vi "test.vi"() -> ()   [LabVIEW 2010, in "Map.lvclass"]
doc: "Test program for the Map class, demonstrating how to use its functionality."
uses:
  Map.lvclass
panel:
  in  "clear button":bool
  in  "delete-element keys":string[](array[string]) caption="key chain"
  in  "delete button":bool
  out "value out":string
  in  "fetch array":bool
  in  "fetch keys":string[](array[string]) caption="key chain"
  in  "insert submap":bool
  in  "insert submap keys":string[](array[string]) caption="key chain"
  in  "insert element":bool
  in  "value in":string
  in  "insert-element keys":string[](array[string]) caption="key chain"
  in  "stop":bool
  in  "elements":string(tree)
  # "Map test program"
  # "The Map class provides the functionality of an associative array, which is a collection of key-value pairs.\n\nYou can address individual elements (values) of a map using a unique key (a string). \n\nAny data type is supported as a value. In this test program only strings and (sub-)Maps are used as values, however.\n\nNested maps (tree-like structures) are possible because a Map can itself be used as a value. You can access values (either submaps or terminal nodes) in the hierarchy by means of key chains (a key chain is an array of strings).\n\nInvidiual elements (nodes) can be added to the tree hierarchy even if parent nodes do not yet exist: just provide a key chain and missing nodes are generated on the fly."
  # "Assign element"
  # "Assign submap"
  # "Fetch element"
  # "Delete element/submap"
  # "Clear map"
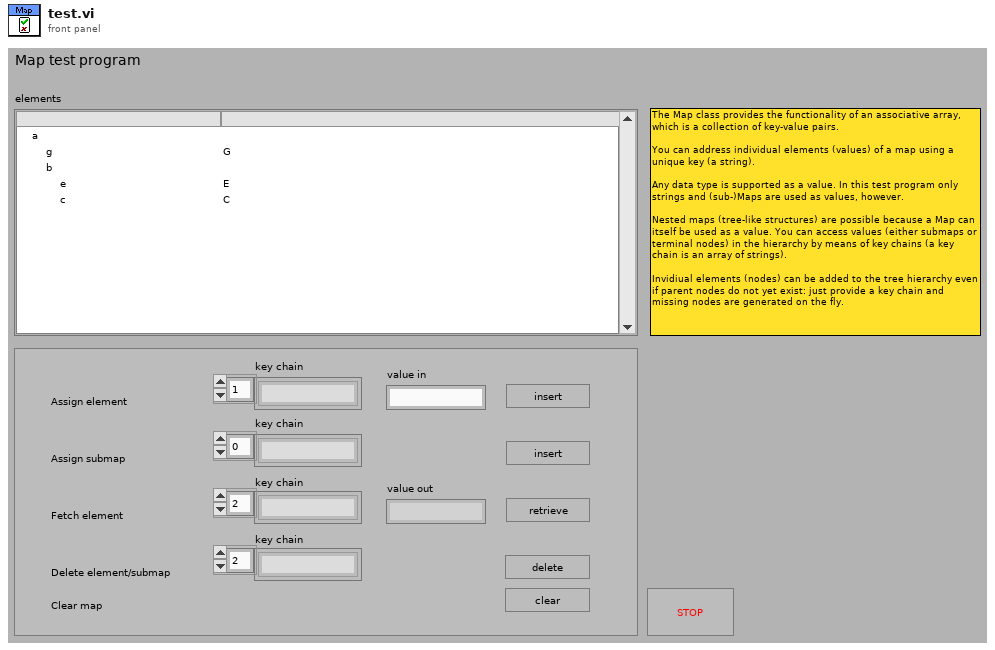
[diagram p1: front panel]
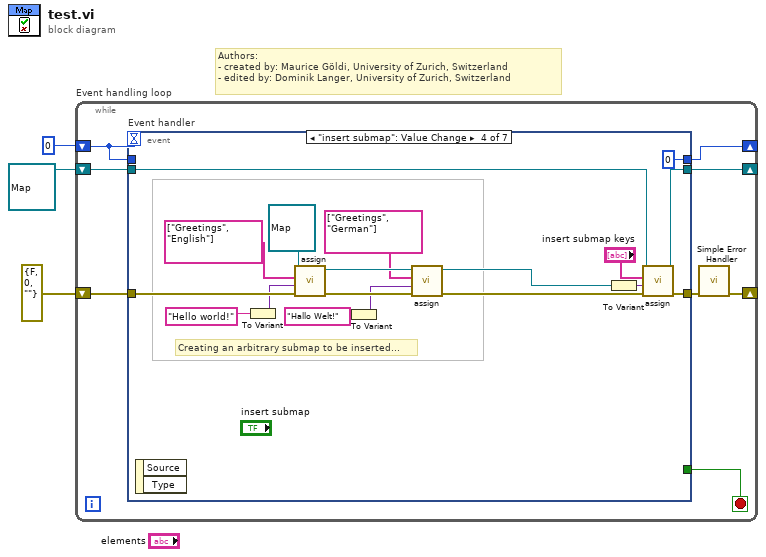
[diagram p0: block diagram]
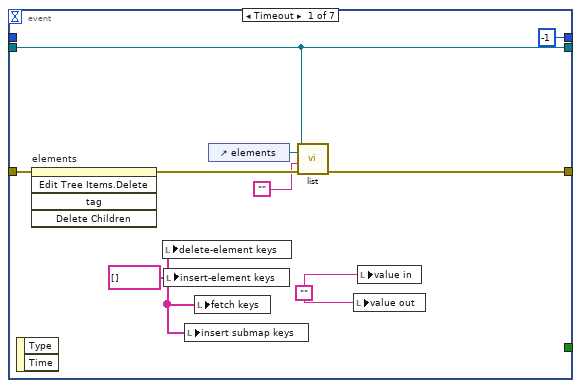
[diagram p2: hidden frame]
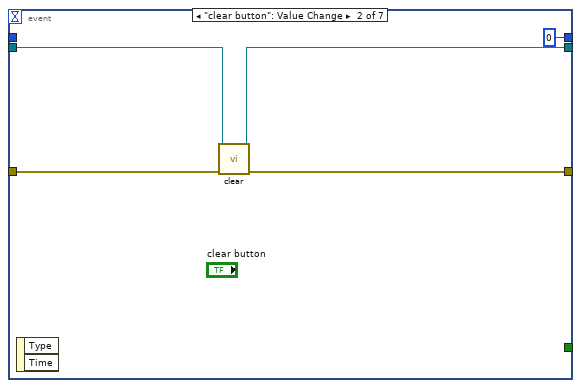
[diagram p3: hidden frame]
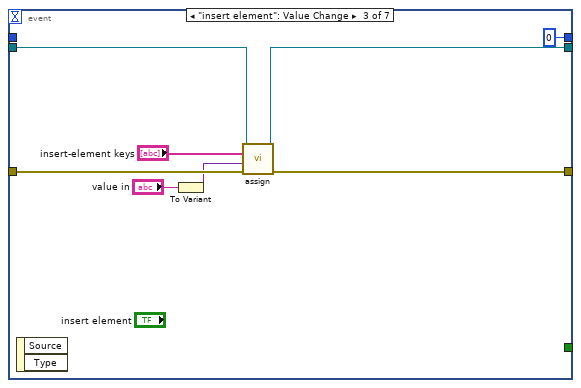
[diagram p4: hidden frame]
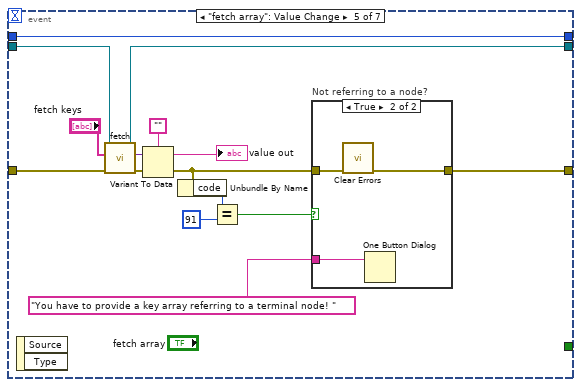
[diagram p5: hidden frame]
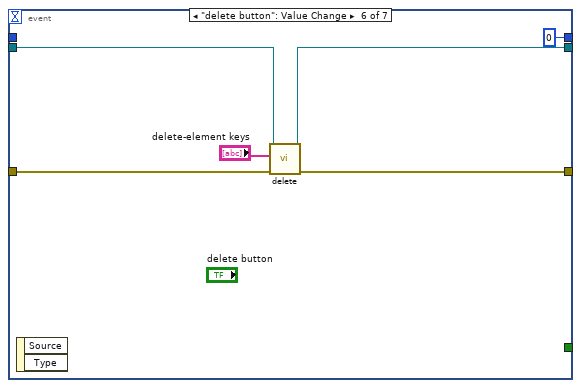
[diagram p7: hidden frame]
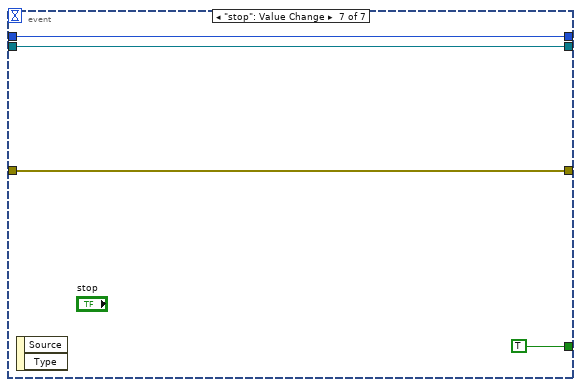
[diagram p8: hidden frame]
diagram:
  # "Authors: \n- created by: Maurice Göldi, University of Zurich, Switzerland\n- edited by: Dominik Langer, University of Zurich, Switzerland"
  n1 = while "Event handling loop" {
    shift-right: [w5] -> _
    shift-left: errorcluster {"status"=FALSE, "code"=0, "source"=""} ("error out") -> [w11]
    shift-right: [w9] -> _
    shift-left: refnum<class "Map.lvclass"> refnum ("Map.lvclass") -> [w10]
    shift-right: [w6] -> _
    shift-left: 0 -> [w7]
    stop <- w8 stop-if-true
    n2 = event "Event handler" shown="[3] \"insert submap\": Value Change" {
      selector: _ -> [_ _ _ _ _ _ _]
      dyn-events: _ -> [_ _ _ _ _ _ _]
      timeout: w7 -> [_ _ _ _ _ _ _]
      tunnel: w11 -> [w19 w25 w31 w51 w65 w75 w80]
      tunnel: [w17 w24 w30 w34 w54 w74 w80] -> w4
      tunnel: w10 -> [w15 w23 w29 w36 w63 w73 w79]
      tunnel: [w15 w22 w28 w35 w62 w72 w79] -> w9
      tunnel: [_ _ _ _ _ _ TRUE] -> w8
      tunnel: w7 -> [_ _ _ _ w66 _ w77]
      tunnel: [-1 0 0 0 w66 0 w77] -> w6
      event Timeout {
        w13 = ""
        w12 = string[] [] ("key array 2")
        n3 = event-data() -> ()  [unwired: 3 out]
        n4 = invoke on="elements" class="Tree (strict)" method="Edit Tree Items.Delete"(error in=w19) -> (error out=w18:errorcluster)  [unwired: 4 in, 4 out]
        n5 = local write "delete-element keys"(w12) -> ()
        n6 = local write "insert-element keys"(w12) -> ()
        n7 = local write "insert submap keys"(w12) -> ()
        n8 = local write "fetch keys"(w12) -> ()
        n9 = control-ref of="elements"() -> (w16:refnum<vi>)
        n10 = call "list.vi"("error in (no error)"=w18, "parent node"="", "tree reference"=w16, "Map in"=w15) -> ("error out"=w17:errorcluster)  [unwired: 7 out]
        n11 = local write "value out"(w13) -> ()
        n12 = local write "value in"(w13) -> ()
      }
      event "clear button": Value Change {
        n13 = event-data() -> ()  [unwired: 3 out]
        n14 = call "clear.vi"("error in (no error)"=w25, "Map in"=w23) -> ("error out"=w24:errorcluster, "Map out"=w22:refnum<class "Map.lvclass">)  [unwired: 8 in]
      }
      event "insert element": Value Change {
        n15 = event-data() -> ()  [unwired: 3 out]
        n16 = To Variant(anything="value in") -> (Variant=w26:variant)
        n17 = call "assign.vi"("error in (no error)"=w31, "value"=w26, "key chain"="insert-element keys", "Map in"=w29) -> ("error out"=w30:errorcluster, "Map out"=w28:refnum<class "Map.lvclass">)  [unwired: 6 in]
      }
      event "insert submap": Value Change {
        # "Creating an arbitrary submap to be inserted..."
        n18 = event-data() -> ()  [unwired: 3 out]
        n19 = To Variant(anything="Hello world!") -> (Variant=w49:variant)
        n20 = call "assign.vi"("error in (no error)"=w51, "value"=w49, "key chain"=string[] ["Greetings", "English"] ("key array"), "Map in"=refnum<class "Map.lvclass"> refnum ("Map.lvclass")) -> ("error out"=w45:errorcluster, "Map out"=w46:refnum<class "Map.lvclass">)  [unwired: 6 in]
        n21 = To Variant(anything="Hallo Welt!") -> (Variant=w44:variant)
        n22 = call "assign.vi"("error in (no error)"=w45, "value"=w44, "key chain"=string[] ["Greetings", "German"] ("key array"), "Map in"=w46) -> ("error out"=w39:errorcluster, "Map out"=w41:refnum<class "Map.lvclass">)  [unwired: 6 in]
        n23 = To Variant(anything=w41) -> (Variant=w38:variant)
        n24 = call "assign.vi"("error in (no error)"=w39, "value"=w38, "key chain"="insert submap keys", "Map in"=w36) -> ("error out"=w34:errorcluster, "Map out"=w35:refnum<class "Map.lvclass">)  [unwired: 6 in]
      }
      event "fetch array": Value Change {
        n25 = event-data() -> ()  [unwired: 3 out]
        n26 = call "fetch.vi"("error in (no error)"=w65, "key chain"="fetch keys", "Map in"=w63) -> ("error out"=w61:errorcluster, "value"=w60:variant, "Map out"=w62:refnum<class "Map.lvclass">)  [unwired: 6 out]
        n27 = Variant To Data(error in=w61, Variant=w60, type="") -> (error out=w55:errorcluster, data=→"value out":string)
        n28 = Unbundle By Name(w55) -> ("code"=w57:i32)
        n29 = Equal?(x=w57, y=91) -> (x = y?=w53:bool)
        n30 = case "Not referring to a node?" shown="True" w53 {
          tunnel: w55 -> [w67 w70]
          tunnel: [w67 w69] -> w54
          tunnel: "You have to provide a key array referring to a terminal node! " ("message") -> [_ w68]
          frame False {
          }
          frame True {
            n31 = call <vilib>:"Clear Errors.vi"("error in (no error)"=w70) -> ("error out"=w69:errorcluster)  [unwired: 6 in]
            n32 = One Button Dialog(message=w68) -> ()  [unwired: 1 in, 1 out]
          }
        }
      }
      event "delete button": Value Change {
        n33 = event-data() -> ()  [unwired: 3 out]
        n34 = call "delete.vi"("error in (no error)"=w75, "key chain"="delete-element keys", "Map in"=w73) -> ("error out"=w74:errorcluster, "Map out"=w72:refnum<class "Map.lvclass">)  [unwired: 7 in]
      }
      event "stop": Value Change {
        n35 = event-data() -> ()  [unwired: 3 out]
      }
    }
    n36 = call <vilib>:"Simple Error Handler.vi"("error in (no error)"=w4) -> ("error out"=w5:errorcluster)  [unwired: 4 in, 4 out]
  }
